vi "Gyro Unwrap Demonstrator.vi"() -> ()   [LabVIEW 2011]
panel:
  out "Output":dbl
  in  "Input":dbl(knob)=180.0 scale=-400.0..400.0
  in  "Modulus":dbl=360.0
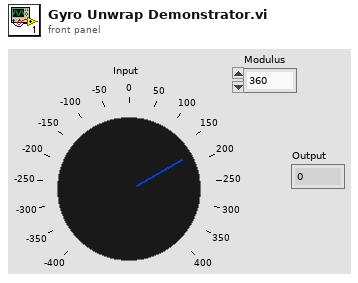
[diagram p1: front panel]
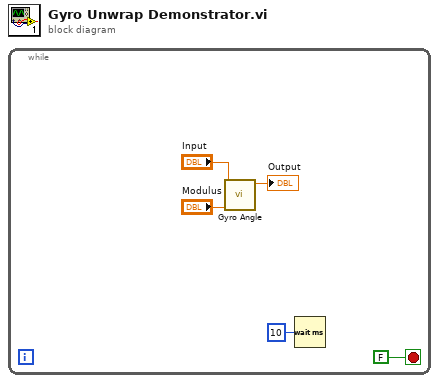
[diagram p0: block diagram]
diagram:
  n1 = while {
    stop <- FALSE stop-if-true
    n2 = call "Gyro Angle.vi"("Mod"="Modulus", "Input"="Input") -> ("Output"=→"Output":dbl)  [unwired: 9 in]
    n3 = Wait (ms)(milliseconds to wait=u32 10) -> ()  [unwired: 1 out]
  }
